vi "Pre-Arm.vi"(8 "error in (no error)":errorcluster, 11 "Lockin Digitizer Driver in":refnum<class "Lockin Digitizer Driver.lvclass">) -> (0 "error out":errorcluster, 3 "Lockin Digitizer Driver out":refnum<class "Lockin Digitizer Driver.lvclass">)   [LabVIEW 2021]
uses:
  Lockin Digitizer Driver.lvclass
panel:
  out "Lock-in channel indexes":i32[](array[numeric])
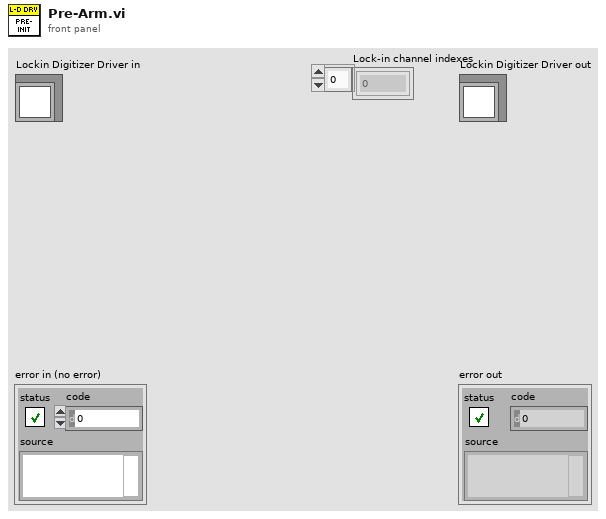
[diagram p1: front panel]
types:
  T1 = typedef "Lockin Digitizer Configuration.ctl" = cluster{"Post-trigger delay":dbl, "Post-trigger duration":dbl, "Rate":dbl, "Ranges":dbl[], "Re-name channels":string[], "Active channels":string, "External\nclock":bool, "Frequencies":dbl[], "Time\nconstant":dbl, "Output \namplitudes":dbl[], "Input\nchannles":string[]}
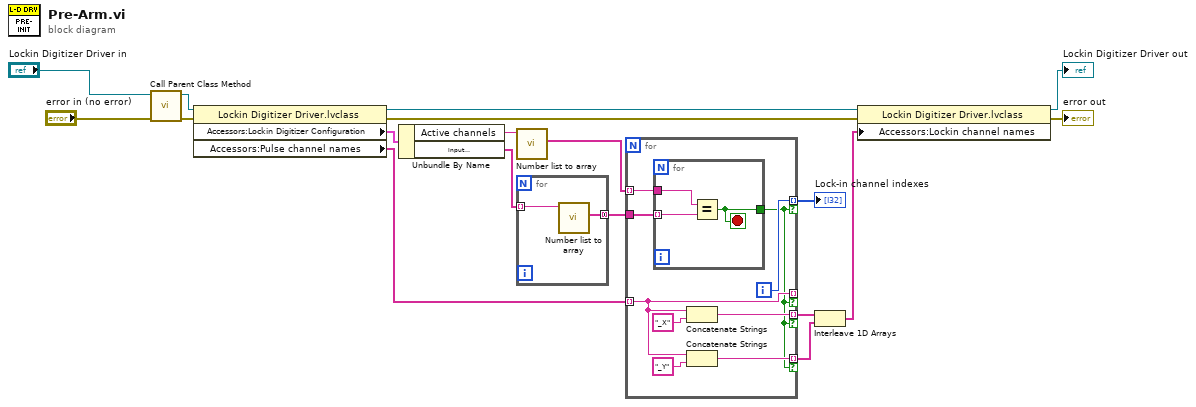
[diagram p0: block diagram]
diagram:
  n1 = call-parent "Call Parent Class Method"("error in (no error)"="error in (no error)", "Pulse Driver in"="Lockin Digitizer Driver in") -> ("error out"=w3:errorcluster, "Pulse Driver out"=w16:refnum<class "Lockin Digitizer Driver.lvclass">)  [unwired: 8 in]
  n2 = property class="Lockin Digitizer Driver.lvclass"(reference=w16, error in=w3) -> (reference out=w8:refnum<class "Lockin Digitizer Driver.lvclass">, error out=w7:errorcluster, "Accessors:Lockin Digitizer Configuration"=w15:T1, "Accessors:Pulse channel names"=w9:string[])
  n3 = Unbundle By Name(w15) -> ("Active channels"=w14:string, "Input\nchannles"=w13:string[])
  n4 = call "Number list to array.vi"("Number list"=w14) -> ("Full names"=w11:string[])  [unwired: 8 in, 2 out]
  n5 = for {
    tunnel: w13 -> [w20] mode=indexing
    tunnel: [w19] -> w12 mode=concatenating
    n6 = call "Number list to array.vi"("Number list"=w20) -> ("Full names"=w19:string[])  [unwired: 8 in, 2 out]
  }
  n7 = for {
    tunnel: w12 -> [w29]
    tunnel: w11 -> [w28] mode=indexing
    tunnel: [w27] -> w10 mode=indexing if=w21
    tunnel: w9 -> [w25] mode=indexing
    tunnel: [w25] -> _ mode=indexing if=w21
    tunnel: [w23] -> w6 mode=indexing if=w21
    tunnel: [w22] -> w5 mode=indexing if=w21
    i -> [w27]
    n8 = for {
      tunnel: w29 -> [w32] mode=indexing
      tunnel: w28 -> [w31]
      tunnel: [w30] -> w21
      stop <- w30 stop-if-true
      n9 = Equal?(x=w31, y=w32) -> (x = y?=w30:bool)
    }
    n10 = Concatenate Strings(w25, "_X" ("string")) -> (w23:string)
    n11 = Concatenate Strings(w25, "_Y" ("string")) -> (w22:string)
  }
  "Lock-in channel indexes" <- w10
  n12 = Interleave 1D Arrays(w6, w5) -> (w4:string[])
  n13 = property class="Lockin Digitizer Driver.lvclass"(reference=w8, error in=w7, "Accessors:Lockin channel names"=w4) -> (reference out=→"Lockin Digitizer Driver out":refnum<class "Lockin Digitizer Driver.lvclass">, error out=→"error out":errorcluster)
